vi "Options GUI.vi"(8 "error in (no error)":errorcluster, 11 "Access Configuration in":T1 {"User array"."Expire sec" format="%.2f"}) -> (0 "error out":errorcluster, 2 "Cancelled?":bool, 3 "Access Configuration out":T1 {"User array"."Expire sec" format="%.2f"})   [LabVIEW 2012]
doc: "This is a pop-up panel which lets the system supervisor either add a new user (if \"New user?\" = T) or edit the existing user with \"Edit index\". It is a modal GUI.\n\nRequired input is the Access Configuration, which contains all the user access configuration parameters and current users.\n\nIf called with \"New user?\" = F the password fields are disabled. If \"New user?\" = T, then the \"Unlock and reset expiration?\" checkbox is not visable. The prompt also changes depending on the state of the \"new user?\" input.\n\nIf a new user, when the supervisor clicks Continue, the code:.\n1) checks that user ID field is not empty\n2) checks that the two new passwords are identical. If not, user is informed and the vi waits for another continue or cancel.\n3) If the two new passwords are equal, they are checked for minimum length of \"Min password char\" (from access configuration cluster) characters. If not of sufficient length, user is informed, and this vi waits for continue or cancel.\n4) the current time is used, along with the \"expire days\" setting from the access configuration cluster, to st the new user's expiration time.\n\nIf NOT a new user, when the supervisor clicks Continue, the code:.\n1) uses \"edit index\" to index the particular user's cluster from the input access configuration.\n2)checks if Active? checkbox is set, and sets corresponding field is user's config cluster.\n3) checks if the supervisor checked the reset checkbox, if set the user's locked and expired fields are cleared and new expiration time is set\n4) copies remaining fields to the user config."
uses:
  User Access Type defs/Continue Button.ctl
  User Access Type defs/Cancel Button.ctl
  User Access Type defs/All users access configuration cluster.ctl
  User Access Type defs/User access cluster array.ctl
  User Access Type defs/User access cluster.ctl
  User Access Type defs/Security level U8.ctl
panel:
  in  "Password Expiration enabled":bool
  in  "Expiration Days":i32=1 min=1 max=99999
  in  "Minimum Password Length":i32=1 min=1 max=99999
  in  "Maximum Password Attempts":i32=3 min=1 max=99999
  in  "Maximum ID Attempts":i32=1 min=1 max=99999
  out "State case":string
  in  "Cancel":T5
  in  "Continue":T6
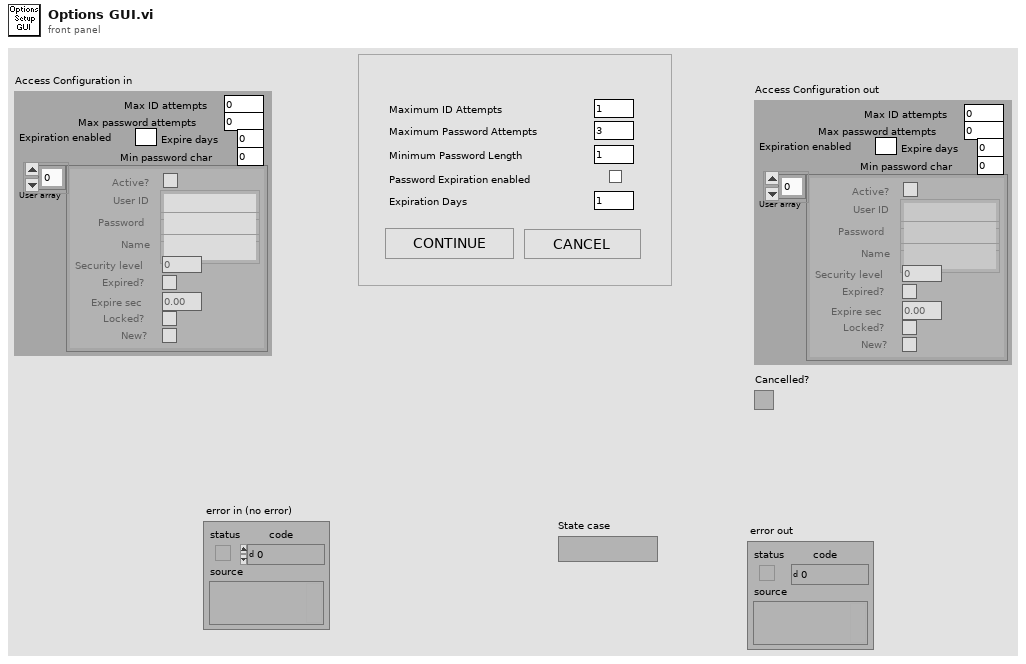
[diagram p1: front panel]
types:
  T1 = typedef "All users access configuration cluster.ctl" = cluster{"Max ID attempts":i32, "Max password attempts":i32, "Expiration enabled":bool, "Expire days":i32, "User array":T2, "Min password char":i32}
  T2 = typedef "User access cluster array.ctl" = T3[]
  T3 = typedef "User access cluster.ctl" = cluster{"Active?":bool, "User ID":string, "Password":string, "Name":string, "Security level":T4, "Expired?":bool, "Expire sec":dbl, "Locked?":bool, "New?":bool}
  T4 = typedef "Security level U8.ctl" = u8
  T5 = typedef "Cancel Button.ctl" = bool
  T6 = typedef "Continue Button.ctl" = bool
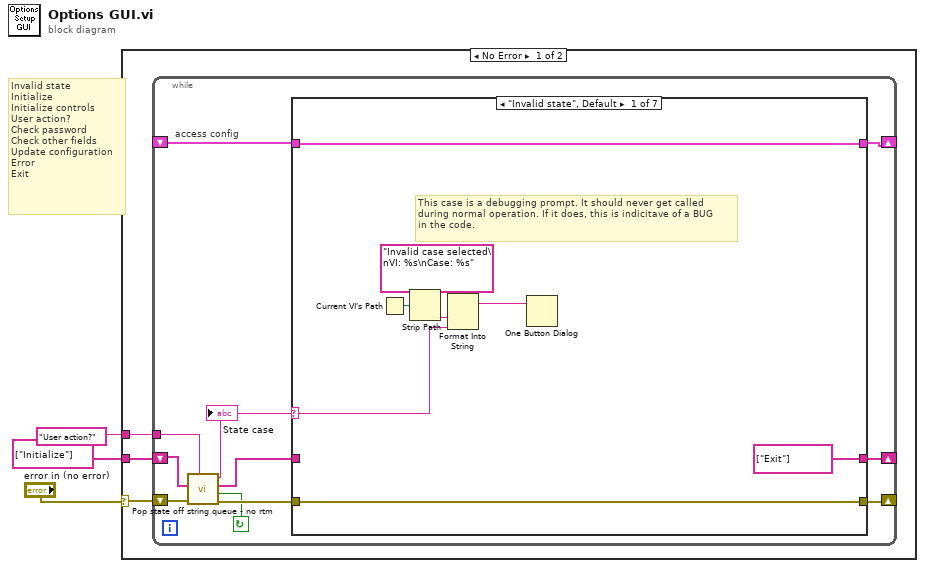
[diagram p0: block diagram]
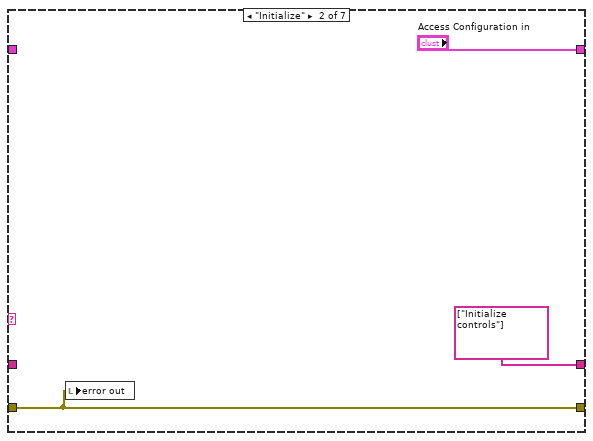
[diagram p2: hidden frame]
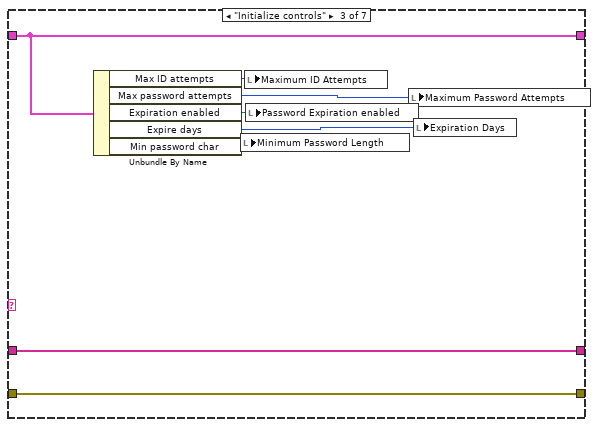
[diagram p3: hidden frame]
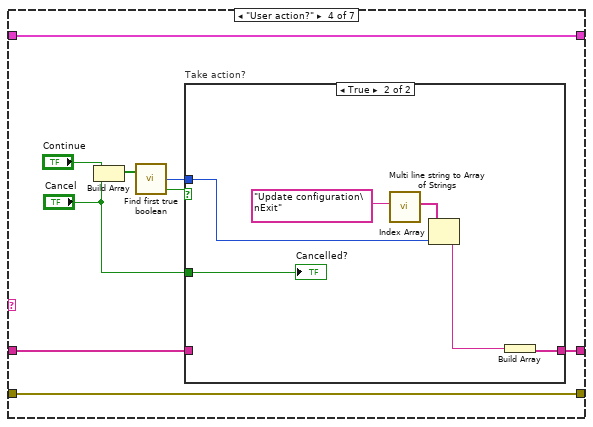
[diagram p4: hidden frame]
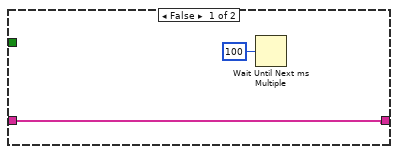
[diagram p5: hidden frame]
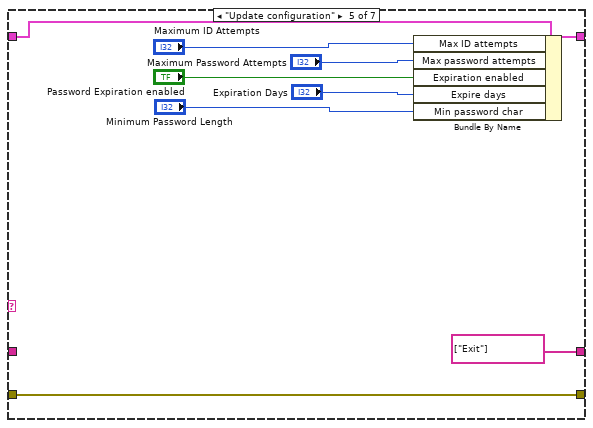
[diagram p6: hidden frame]
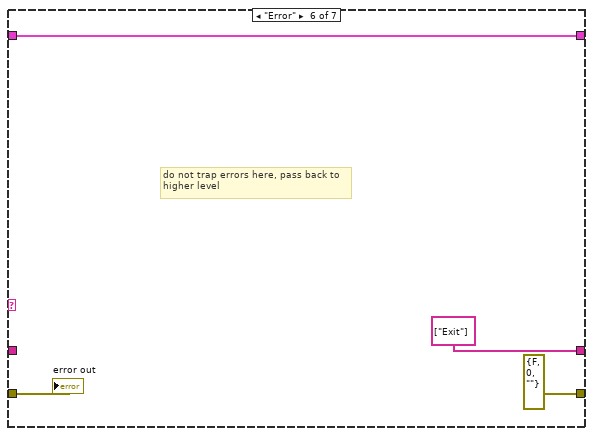
[diagram p7: hidden frame]
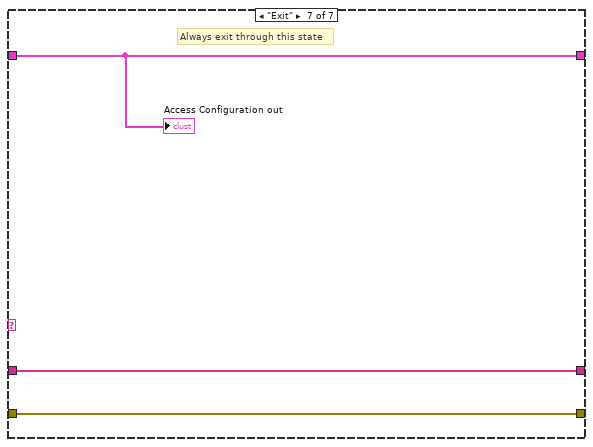
[diagram p8: hidden frame]
diagram:
  # "Invalid state\nInitialize\nInitialize controls\nUser action?\nCheck password\nCheck other fields\nUpdate configuration\nError\nExit"
  n1 = case shown="No Error" "error in (no error)" {
    selector: "error in (no error)" -> [w6 _]
    tunnel: string[] ["Initialize"] ("State que out") -> [w5 _]
    tunnel: "User action?" ("Default state") -> [w4 _]
    frame No Error {
      n2 = while {
        tunnel: w4 -> [w9]
        shift-left: w5 -> [w13]
        shift-right: [w11] -> _
        shift-left: w6 -> [w17]
        shift-right: [w15] -> _
        shift-right: [w7] -> _
        shift-left: _ -> [w8]
        stop <- w10 continue-if-true
        # "access config"
        n3 = call "Pop state off string queue - no rtm.vi"("Default state"=w9, "error in (no error)"=w17, "State que in"=w13) -> ("error out"=w16:errorcluster, "Not Exit?"=w10:bool, "State que out"=w12:string[], "State case"=w14:string)  [unwired: 5 out]
        "State case" <- w14
        n4 = case shown="\"Invalid state\", Default" w14 {
          selector: w14 -> [w20 _ _ _ _ _ _]
          tunnel: [w25 w28 w36 w45 w59 errorcluster {"status"=FALSE, "code"=0, "source"=""} ("error out") w68] -> w15
          tunnel: w16 -> [w25 w28 w36 w45 w59 w64 w68]
          tunnel: [string[] ["Exit"] ("State que out") string[] ["Initialize controls"] ("State que out") w35 w44 string[] ["Exit"] ("State que out") string[] ["Exit"] ("State que out") w69] -> w11
          tunnel: w12 -> [_ _ w35 w38 _ _ w69]
          tunnel: [w18 "Access Configuration in" w34 w43 w60 w63 w67] -> w7
          tunnel: w8 -> [w18 _ w34 w43 w61 w63 w67]
          frame "Invalid state", Default {
            # "This case is a debugging prompt. It should never get called\nduring normal operation. If it does, this is indicitave of a BUG\nin the code."
            n5 = Current VI's Path() -> (path=w22:path)
            n6 = Strip Path(path=w22) -> (name=w21:string)  [unwired: 1 out]
            n7 = Format Into String(format string="Invalid case selected\nVI: %s\nCase: %s" ("message"), w21, w20) -> (resulting string=w23:string)  [unwired: 2 in, 1 out]
            n8 = One Button Dialog(message=w23) -> ()  [unwired: 2 out]
          }
          frame "Initialize" {
            n9 = local write "error out"(w28) -> ()
          }
          frame "Initialize controls" {
            n10 = Unbundle By Name(w34) -> ("Max ID attempts"=w33:i32, "Max password attempts"=w29:i32, "Expiration enabled"=w30:bool, "Expire days"=w31:i32, "Min password char"=w32:i32)
            n11 = local write "Minimum Password Length"(w32) -> ()
            n12 = local write "Maximum ID Attempts"(w33) -> ()
            n13 = local write "Password Expiration enabled"(w30) -> ()
            n14 = local write "Maximum Password Attempts"(w29) -> ()
            n15 = local write "Expiration Days"(w31) -> ()
          }
          frame "User action?" {
            n16 = Build Array("Continue", "Cancel") -> (w41:T5[])
            n17 = call "Find first true boolean.vi"("Boolean Array IN"=w41) -> ("Index of first (T)"=w39:i32, "True found?"=w40:bool)  [unwired: 2 out]
            n18 = case "Take action?" shown="True" w40 {
              tunnel: [w47 w50] -> w44
              tunnel: w39 -> [_ w52]
              tunnel: w38 -> [w47 _]
              tunnel: "Cancel" -> [_ w49]
              frame False {
                n19 = Wait Until Next ms Multiple(millisecond multiple=u32 100) -> ()  [unwired: 1 out]
              }
              frame True {
                n20 = call "Multi line string to Array of Strings.vi"("Multi Line String"="Update configuration\nExit") -> ("Array of Strings"=w53:string[])  [unwired: 6 out]
                n21 = Index Array(array=w53, index=w52) -> (element=w51:string)
                n22 = Build Array(w51) -> (w50:string[])
                "Cancelled?" <- w49
              }
            }
          }
          frame "Update configuration" {
            n23 = Bundle By Name(cluster=w61, "Max ID attempts"="Maximum ID Attempts", "Max password attempts"="Maximum Password Attempts", "Expiration enabled"="Password Expiration enabled", "Expire days"="Expiration Days", "Min password char"="Minimum Password Length") -> (w60:T1)
          }
          frame "Error" {
            # "do not trap errors here, pass back to\nhigher level"
            "error out" <- w64
          }
          frame "Exit" {
            # "Always exit through this state"
            "Access Configuration out" <- w67
          }
        }
      }
    }
    frame Error {
    }
  }
